vi "Report Event or Error.vi"(5 "Severity Code (error)":T1=enum."error", 7 "Facility Code (user)":T2=enum."user", 8 "error in (no error)":errorcluster, 9 "Message Content":string, 10 "Message Tag":string, 11 "Logger.syslog in":refnum<class "Logger.syslog.lvclass">) -> (0 "error out":errorcluster, 3 "Logger.syslog out":refnum<class "Logger.syslog.lvclass">)   [LabVIEW 2019, in "Logger.syslog.lvlib" / "Logger.syslog.lvclass"]
uses:
  Logger.syslog.lvclass
  <vilib>/NI/syslog/_subVIs/TypeDefs/syslog_facility_codes.ctl
  <vilib>/NI/syslog/_subVIs/TypeDefs/syslog_severity_codes.ctl
panel:
  out "parsed message (what gets logged)":string
  out "Syslog Message":string
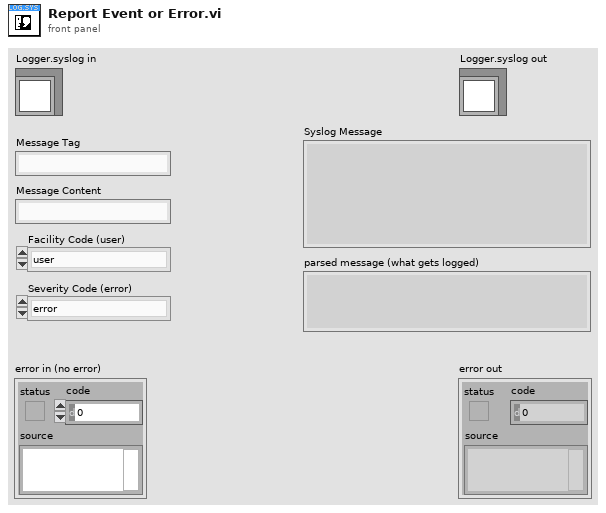
[diagram p1: front panel]
types:
  T1 = typedef "syslog_severity_codes.ctl" = enum16{"emergency", "alert", "critical", "error", "warning", "notice", "info", "debug"}
  T2 = typedef "syslog_facility_codes.ctl" = enum16{"kernel", "user", "mail", "system daemons", "security/authorization", "syslogd", "line printer", "network news", "uucp", "clock daemon", "security/authorization (alternate)", "FTP daemon", "NTP subsystem", "log audit", "log alert", "clock daemon (alternate)", "local use 0", "local use 1", "local use 2", "local use 3", "local use 4", "local use 5", "local use 6", "local use 7"}
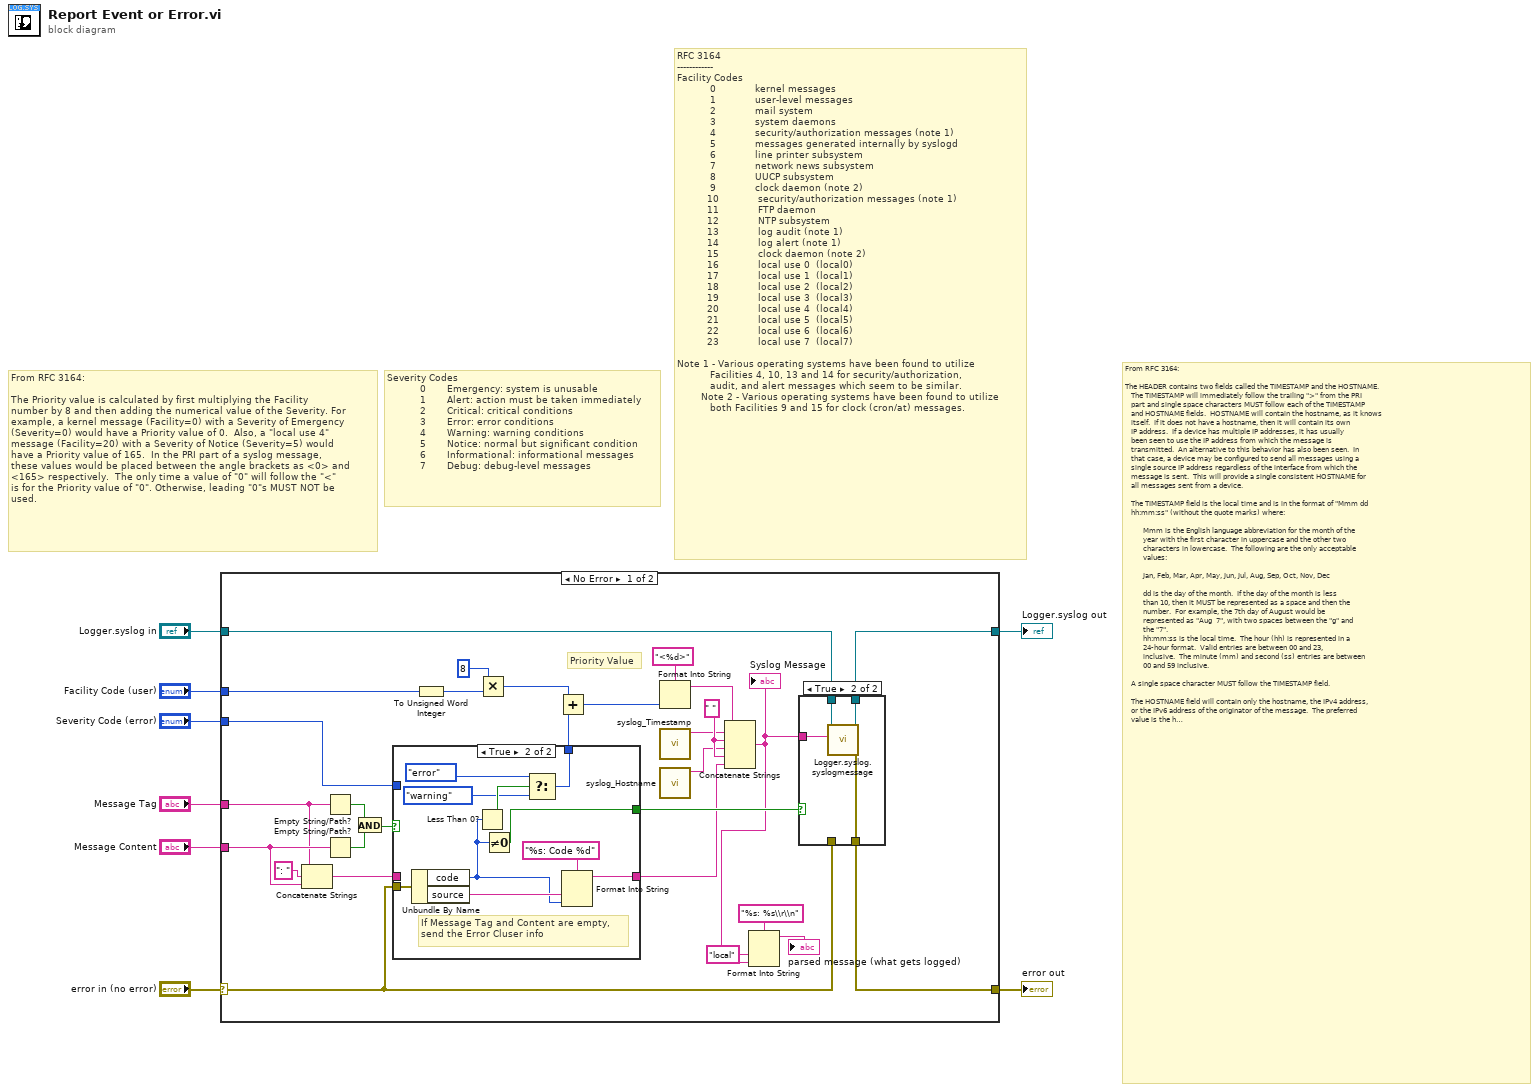
[diagram p0: block diagram]
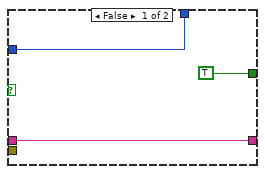
[diagram p3: hidden frame]
diagram:
  # "Severity Codes\n           0       Emergency: system is unusable\n           1       Alert: action must be taken immediately\n           2       Critical: critical conditions\n           3       Error: error conditions\n           4       Warning: warning conditions\n           5       Notice: normal but significant condition\n           6       Informational: informational messages\n           7       Debug: debug-level messages"
  # "RFC 3164\n------------  \nFacility Codes\n           0             kernel messages\n           1             user-level messages\n           2             mail system\n           3             system daemons\n           4             security/authorization messages (note 1)\n           5             messages generated internally by syslogd\n           6             line printer subsystem\n           7             network news subsystem\n           8             UUCP subsystem\n           9             clock daemon (note 2)\n          10             security/authorization messages (note 1)\n          11             FTP daemon\n          12             NTP subsystem\n          13             log audit (note 1)\n          14             log alert (note 1)\n          15             clock daemon (note 2)\n          16             local use 0  (local0)\n          17             local use 1  (local1)\n          18             local use 2  (local2)\n          19             local use 3  (local3)\n          20             local use 4  (local4)\n          21             local use 5  (local5)\n          22             local use 6  (local6)\n          23             local use 7  (local7)\n\nNote 1 - Various operating systems have been found to utilize\n           Facilities 4, 10, 13 and 14 for security/authorization,\n           audit, and alert messages which seem to be similar.\n        Note 2 - Various operating systems have been found to utilize\n           both Facilities 9 and 15 for clock (cron/at) messages."
  # "From RFC 3164:\n\nThe HEADER contains two fields called the TIMESTAMP and the HOSTNAME.\n   The TIMESTAMP will immediately follow the trailing \">\" from the PRI\n   part and single space characters MUST follow each of the TIMESTAMP\n   and HOSTNAME fields.  HOSTNAME will contain the hostname, as it knows\n   itself.  If it does not have a hostname, then it will contain its own\n   IP address.  If a device has multiple IP addresses, it has usually\n   been seen to use the IP address from which the message is\n   transmitted.  An alternative to this behavior has also been seen.  In\n   that case, a device may be configured to send all messages using a\n   single source IP address regardless of the interface from which the\n   message is sent.  This will provide a single consistent HOSTNAME for\n   all messages sent from a device.\n\n   The TIMESTAMP field is the local time and is in the format of \"Mmm dd\n   hh:mm:ss\" (without the quote marks) where:\n\n         Mmm is the English language abbreviation for the month of the\n         year with the first character in uppercase and the other two\n         characters in lowercase.  The following are the only acceptable\n         values:\n\n         Jan, Feb, Mar, Apr, May, Jun, Jul, Aug, Sep, Oct, Nov, Dec\n\n         dd is the day of the month.  If the day of the month is less\n         than 10, then it MUST be represented as a space and then the\n         number.  For example, the 7th day of August would be\n         represented as \"Aug  7\", with two spaces between the \"g\" and\n         the \"7\".\n         hh:mm:ss is the local time.  The hour (hh) is represented in a\n         24-hour format.  Valid entries are between 00 and 23,\n         inclusive.  The minute (mm) and second (ss) entries are between\n         00 and 59 inclusive.\n\n   A single space character MUST follow the TIMESTAMP field.\n\n   The HOSTNAME field will contain only the hostname, the IPv4 address,\n   or the IPv6 address of the originator of the message.  The preferred\n   value is the hostname.  If the hostname is used, the HOSTNAME field\n   MUST contain the hostname of the device as specified in STD 13 [4].\n   It should be noted that this MUST NOT contain any embedded spaces.\n   The Domain Name MUST NOT be included in the HOSTNAME field.  If the\n   IPv4 address is used, it MUST be shown as the dotted decimal notation\n   as used in STD 13 [5].  If an IPv6 address is used, any valid\n   representation used in RFC 2373 [6] MAY be used.  A single space\n   character MUST also follow the HOSTNAME field."
  # "From RFC 3164:\n\nThe Priority value is calculated by first multiplying the Facility\nnumber by 8 and then adding the numerical value of the Severity. For\nexample, a kernel message (Facility=0) with a Severity of Emergency\n(Severity=0) would have a Priority value of 0.  Also, a \"local use 4\"\nmessage (Facility=20) with a Severity of Notice (Severity=5) would\nhave a Priority value of 165.  In the PRI part of a syslog message,\nthese values would be placed between the angle brackets as <0> and\n<165> respectively.  The only time a value of \"0\" will follow the \"<\"\nis for the Priority value of \"0\". Otherwise, leading \"0\"s MUST NOT be\nused."
  n1 = case shown="No Error" "error in (no error)" {
    selector: "error in (no error)" -> [w14 w58]
    tunnel: [w15 w58] -> w7
    tunnel: [w16 w57] -> w5
    tunnel: "Logger.syslog in" -> [w17 w57]
    tunnel: "Severity Code (error)" -> [w22 _]
    tunnel: "Facility Code (user)" -> [w21 _]
    tunnel: "Message Content" -> [w20 _]
    tunnel: "Message Tag" -> [w19 _]
    frame No Error {
      w29 = " " ("string")
      # "Priority Value"
      n2 = Concatenate Strings(w19, ": " ("string"), w20) -> (w34:string)
      n3 = Empty String/Path?(string/path=w19) -> (empty?=w31:bool)
      n4 = Empty String/Path?(string/path=w20) -> (empty?=w32:bool)
      n5 = And(x=w31, y=w32) -> (x .and. y?=w30:bool)
      n6 = case shown="True" w30 {
        tunnel: [w45 w55] -> w12
        tunnel: [TRUE ("status") w54] -> w18
        tunnel: w34 -> [w45 _]
        tunnel: [w44 w50] -> w26
        tunnel: w14 -> [_ w49]
        tunnel: w22 -> [w44 _]
        frame False {
        }
        frame True {
          # "If Message Tag and Content are empty,\nsend the Error Cluser info"
          n7 = Unbundle By Name(w49) -> ("code"=w47:i32, "source"=w48:string)
          n8 = Less Than 0?(x=w47) -> (x < 0?=w53:bool)
          n9 = Not Equal To 0?(x=w47) -> (x != 0?=w54:bool)
          n10 = Select(t=syslog_severity_codes."error" ("Severity (error)"), s=w53, f=syslog_severity_codes."warning") -> (s? t:f=w50:T1)
          n11 = Format Into String(format string="%s: Code %d", w48, w47) -> (resulting string=w55:string)  [unwired: 2 in, 1 out]
        }
      }
      n12 = To Unsigned Word Integer(number=w21) -> (unsigned 16bit integer=w35:u16)
      n13 = Multiply(x=u16 8, y=w35) -> (x*y=w37:u16)
      n14 = Add(x=w37, y=w26) -> (x+y=w25:u16)
      n15 = Format Into String(format string="<%d>", w25) -> (resulting string=w24:string)  [unwired: 2 in, 1 out]
      n16 = call <vilib>:"syslog_Timestamp.vi"() -> ("Timestamp"=w28:string)  [unwired: 11 in]
      n17 = call <vilib>:"syslog_Hostname.vi"() -> ("Hostname"=w27:string)  [unwired: 11 in]
      n18 = Concatenate Strings(w24, w28, w29, w27, w29, w12) -> (w11:string)
      "Syslog Message" <- w11
      n19 = Format Into String(format string="%s: %s\\r\\n" ("string"), "local" ("input 1"), w11) -> (resulting string=→"parsed message (what gets logged)":string)  [unwired: 2 in, 1 out]
      n20 = case shown="True" w18 {
        tunnel: [w38 w43] -> w15
        tunnel: w17 -> [w39 w42]
        tunnel: w11 -> [_ w41]
        tunnel: [w39 w40] -> w16
        tunnel: w14 -> [w38 _]
        frame False {
        }
        frame True {
          n21 = call "Logger.syslog.syslogmessage.vi"("syslog message"=w41, "Logger.syslog"=w42) -> ("error out"=w43:errorcluster, "Logger.syslog out"=w40:refnum<class "Logger.syslog.lvclass">)  [unwired: 8 in]
        }
      }
    }
    frame Error {
    }
  }
  "error out" <- w7
  "Logger.syslog out" <- w5
